vi "Get Auxilary Data.vi"(8 "error in":errorcluster, 11 "Neph in":refnum<class "Nephelometer.lvclass">) -> (0 "error out":errorcluster, 2 "Auxilary data":T1, 3 "Neph out":refnum<class "Nephelometer.lvclass">)   [LabVIEW 2014, in "Nephelometer.lvclass"]
uses:
  Nephelometer.lvclass
  Nephelometer.lvclass/Nephelometer.ctl
  Reusable/Session APIs/Serial/Public/Get Data/Get String.vi
  Reusable/Session APIs/Text Communication/Text Device Session.lvclass
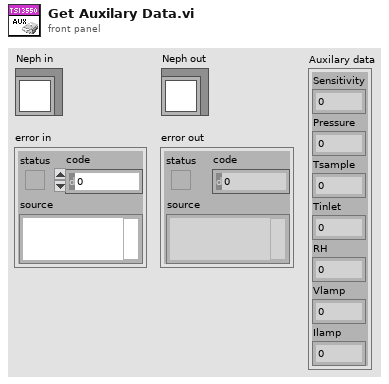
[diagram p1: front panel]
types:
  T1 = cluster{"Sensitivity":dbl, "Pressure":dbl, "Tsample":dbl, "Tinlet":dbl, "RH":dbl, "Vlamp":dbl, "Ilamp":dbl}
  T2 = typedef "Session - Root.lvclass/Session Handle.ctl" = refnum<data-value>
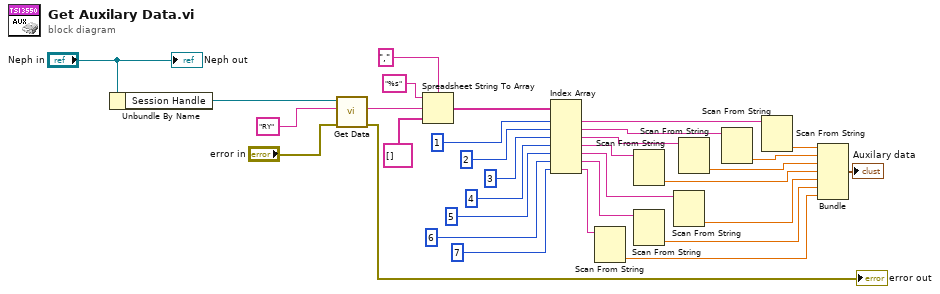
[diagram p0: block diagram]
diagram:
  n1 = Unbundle By Name("Neph in") -> ("Session Handle"=w1:T2)
  n2 = call-poly "Get Data.vi"("error in"="error in", "CMD"="RY", "handle in"=w1) -> ("error out"=→"error out":errorcluster, "DataOut"=w5:string)  [unwired: 6 in, 1 out]
  n3 = Spreadsheet String To Array(delimiter (Tab)=",", format string="%s", spreadsheet string=w5, array type (2D Dbl)=string[] []) -> (array=w28:string[])
  n4 = Index Array(array=w28, index #1=1 ("index"), index #2=2 ("index"), index #3=3 ("index"), index #4=4 ("index"), index #5=5 ("index"), index #6=6 ("index"), index #7=7 ("index")) -> (element #1=w26:string, element #2=w23:string, element #3=w20:string, element #4=w18:string, element #5=w14:string, element #6=w10:string, element #7=w8:string)
  n5 = Scan From String(input string=w8) -> (output 1=w7:dbl)  [unwired: 4 in, 3 out]
  n6 = Scan From String(input string=w18) -> (output 1=w16:dbl)  [unwired: 4 in, 3 out]
  n7 = Scan From String(input string=w10) -> (output 1=w9:dbl)  [unwired: 4 in, 3 out]
  n8 = Scan From String(input string=w14) -> (output 1=w13:dbl)  [unwired: 4 in, 3 out]
  n9 = Scan From String(input string=w20) -> (output 1=w19:dbl)  [unwired: 4 in, 3 out]
  n10 = Scan From String(input string=w23) -> (output 1=w22:dbl)  [unwired: 4 in, 3 out]
  n11 = Scan From String(input string=w26) -> (output 1=w25:dbl)  [unwired: 4 in, 3 out]
  n12 = Bundle(w25, w22, w19, w16, w13, w9, w7) -> (→"Auxilary data":cluster{dbl, dbl, dbl, dbl, dbl, dbl, dbl})  [unwired: 1 in]
  "Neph out" <- "Neph in"
